vi "Read.vi"(8 "error in (no error)":errorcluster, 11 "TDMS Channel in":refnum<class "Channel.lvclass">) -> (0 "error out":errorcluster, 1 "Channel Properties":refnum<class "Variant.lvclass">, 2 "Data":refnum<class "Generic Data.lvclass">, 3 "Channel Name":string)   [LabVIEW 2020, in "TDMS.lvlib" / "Channel.lvclass"]
doc: "Read Channel Name, Data and Properties."
uses:
  Channel.lvclass
  PPL/HDH.Data.Generic.lvlibp/Generic Data/Generic Data.lvclass
  PPL/HDH.Data.Generic.lvlibp/Generic Data/Variant/Variant.lvclass
  Channel.lvclass/Channel.ctl
  PPL/HDH.Data.Generic.lvlibp/Generic Data/Generic Array Data/Generic Array Data.lvclass
  C:/Current projects/WS/PPL/HDH.Data.Generic.lvlibp/Generic Data/Generic Data.lvclass
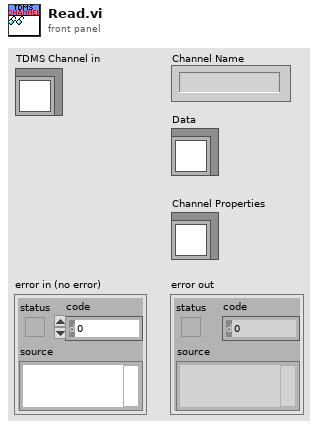
[diagram p1: front panel]
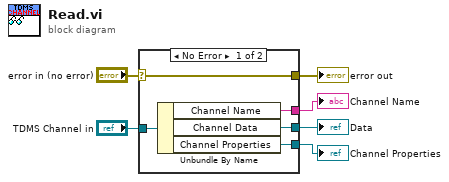
[diagram p0: block diagram]
diagram:
  n1 = case shown="No Error" "error in (no error)" {
    selector: "error in (no error)" -> [w11 w12]
    tunnel: [w11 w12] -> w5
    tunnel: "TDMS Channel in" -> [w10 _]
    tunnel: [w9 _] -> w3
    tunnel: [w8 _] -> w2
    tunnel: [w7 _] -> w1
    frame No Error {
      n2 = Unbundle By Name(w10) -> ("Channel Name"=w9:string, "Channel Data"=w8:refnum<class "Generic Array Data.lvclass">, "Channel Properties"=w7:refnum<class "Variant.lvclass">)
    }
    frame Error {
    }
  }
  "error out" <- w5
  "Channel Name" <- w3
  "Data" <- w2
  "Channel Properties" <- w1
